vi "StopMovement Core.vi"(8 "error in (no error)":errorcluster, 10 "AxisNumber":u8, 11 "CS++SimMotor in":refnum<class "CS++SimMotor.lvclass">) -> (0 "error out":errorcluster, 3 "CS++SimMotor out":refnum<class "CS++SimMotor.lvclass">)   [LabVIEW 2015, in "CS++SimMotor.lvlib" / "CS++SimMotor.lvclass"]
doc: "Stops the movement of an axis."
uses:
  CS++SimMotor.lvclass
  CS++SimMotor.lvclass/CS++SimMotor.ctl
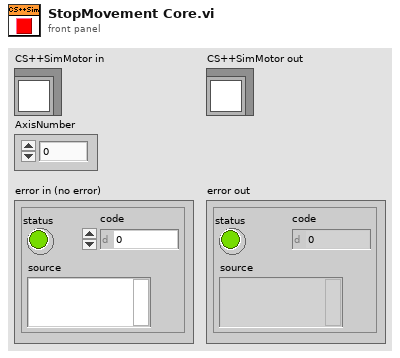
[diagram p1: front panel]
types:
  T1 = enum16{"RelativeMovement", "AbsoluteMovement", "Stop", "ReferenceMovement"}
  T2 = cluster{"AxisNumber":u8, dbl, "Enum":enum16{"RelativeMovement", "AbsoluteMovement", "Stop", "ReferenceMovement"}}
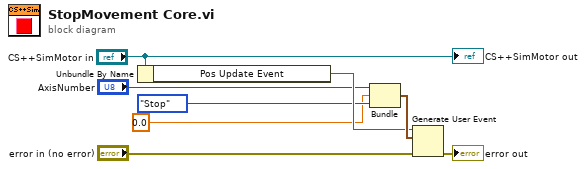
[diagram p0: block diagram]
diagram:
  n1 = Unbundle By Name("CS++SimMotor in") -> ("Pos Update Event"=w7:refnum<user-event>)
  n2 = Bundle("AxisNumber"="AxisNumber", 0.0, "Enum"=T1."Stop") -> (w8:T2)  [unwired: 1 in]
  n3 = Generate User Event(user event=w7, event data cluster=w8, error in="error in (no error)") -> (error out=→"error out":errorcluster)  [unwired: 1 in, 1 out]
  "CS++SimMotor out" <- "CS++SimMotor in"
